vi "QCA - DUT Abort Transmit.vi"(0 "CART TCP Connection In":refnum<k5>, 11 "error in (no error)":errorcluster) -> (4 "CART TCP Connection Out":refnum<k5>, 8 "TCP Messages":string[](array[string]), 15 "error out":errorcluster)   [LabVIEW 2011]
uses:
  Controls/Parameter.ctl
  NART Constants.vi
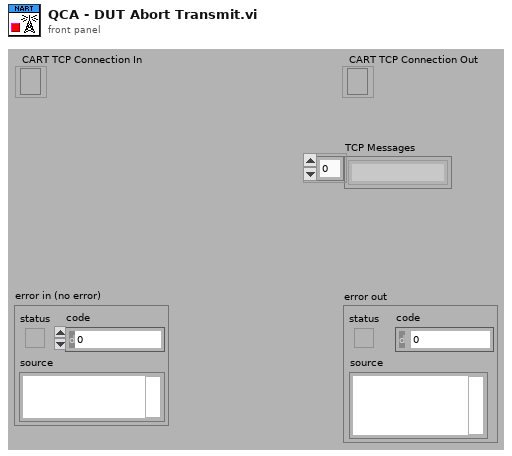
[diagram p1: front panel]
types:
  T1 = typedef "Parameter.ctl" = cluster{"Name":string, "Type":enum16{"decimal", "string", "float", "hex"}}
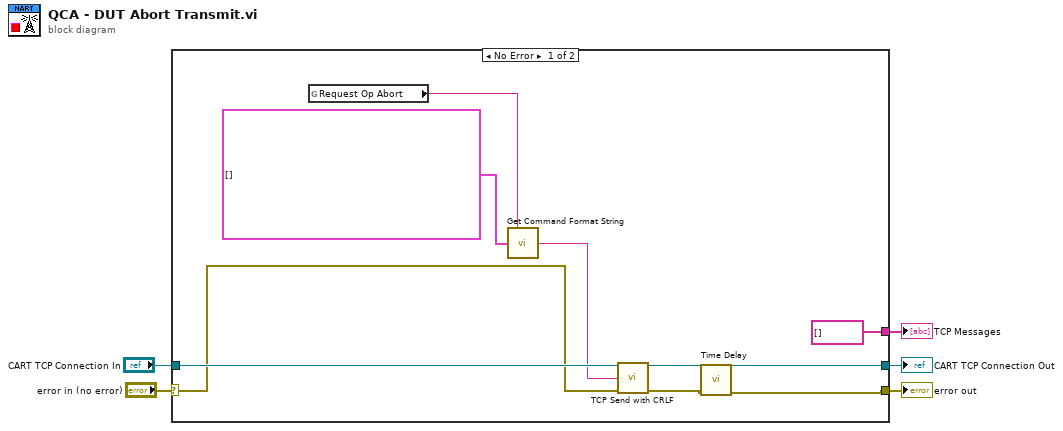
[diagram p0: block diagram]
diagram:
  n1 = case shown="No Error" "error in (no error)" {
    selector: "error in (no error)" -> [w11 w16]
    tunnel: [w6 w16] -> w4
    tunnel: "CART TCP Connection In" -> [w14 w15]
    tunnel: [w10 w15] -> w2
    tunnel: [string[] [] ("TCP Messages") _] -> w1
    frame No Error {
      n2 = global read "NART Constants.vi" "Request Op Abort"() -> (w9:string)
      n3 = call "Get Command Format String.vi"("Command"=w9, "Parameters"=T1[] []) -> ("Command Format String"=w12:string)  [unwired: 13 in]
      n4 = call "TCP Send with CRLF.vi"("CART TCP Connection"=w14, "data in"=w12, "error IO"=w11) -> ("CART TCP Connection Out"=w10:refnum<k5>, "error out"=w7:errorcluster)  [unwired: 11 in]
      n5 = call "Time Delay"("error in (no error)"=w7) -> ("error out"=w6:errorcluster)  [unwired: 10 in]
    }
    frame Error {
    }
  }
  "error out" <- w4
  "CART TCP Connection Out" <- w2
  "TCP Messages" <- w1
